vi "Read waiting measurements launch queue.vi"(8 "error in (no error)":errorcluster, 11 "Controller in":refnum<class "Controller.lvclass">) -> (0 "error out":errorcluster, 2 "stack of waiting msmt requests":refnum<class "Launch Measurements Message.lvclass">[](array[class]), 3 "Controller out":refnum<class "Controller.lvclass">)   [LabVIEW 2016, in "Controller Actor.lvlib" / "Controller.lvclass"]
uses:
  Controller.lvclass
  Messages/Launch Measurements Message/Launch Measurements Message.lvclass
  Controller.lvclass/Controller.ctl
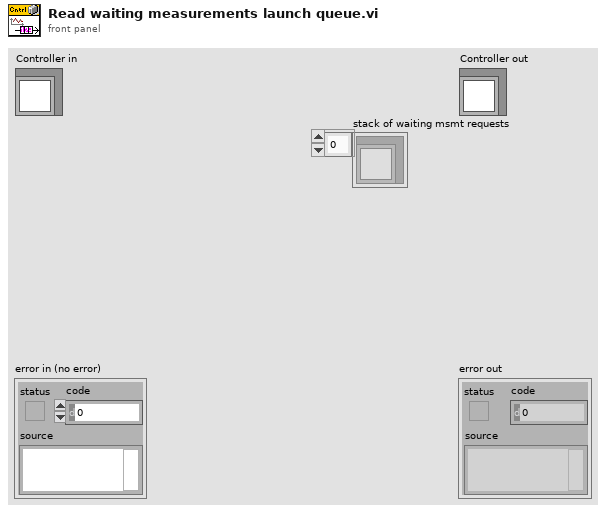
[diagram p1: front panel]
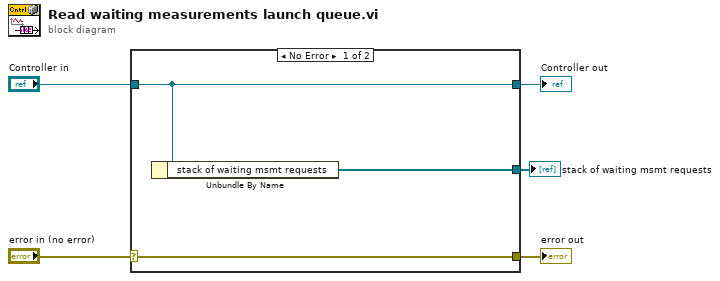
[diagram p0: block diagram]
diagram:
  n1 = case shown="No Error" "error in (no error)" {
    selector: "error in (no error)" -> [w8 w9]
    tunnel: [w8 w9] -> w4
    tunnel: [w7 w10] -> w2
    tunnel: "Controller in" -> [w7 w10]
    tunnel: [w6 _] -> w1
    frame No Error {
      n2 = Unbundle By Name(w7) -> ("stack of waiting msmt requests"=w6:refnum<class "Launch Measurements Message.lvclass">[])
    }
    frame Error {
    }
  }
  "error out" <- w4
  "Controller out" <- w2
  "stack of waiting msmt requests" <- w1
